vi "do_gsw_step.vi"(6 "Optimisation Resolution":i32, 7 "Sinc Zero":dbl, 11 "Spots In":T1[](array[typedef]) {"Amplitude Correction" step=0.1; "Line Trapping"."Phase Gradient" step=0.05; "Line Trapping"."Vector"."x" step=1e-06 format="%#_6p"; "Line Trapping"."Vector"."y" step=1e-06 format="%#_6p"; "Line Trapping"."Vector"."z" step=1e-06 format="%#_6p"; "NA Position"."r" step=1e-06; "NA Position"."y" step=1e-06; "NA Position"."x" step=1e-06; "Position"."z" step=1e-06; "Position"."y" step=1e-06; "Position"."x" step=1e-06; "Phase" step=0.7753; "Intensity" step=0.1}) -> (1 "non-uniformity":dbl=0.056229799277855076 format="%0.2f", 2 "efficiency":dbl=0.953044464704264, 3 "Spots Out":T1[](array[typedef]) {"Amplitude Correction" step=0.1; "Line Trapping"."Phase Gradient" step=0.05; "Line Trapping"."Vector"."x" step=1e-06 format="%#_6p"; "Line Trapping"."Vector"."y" step=1e-06 format="%#_6p"; "Line Trapping"."Vector"."z" step=1e-06 format="%#_6p"; "NA Position"."r" step=1e-06; "NA Position"."y" step=1e-06; "NA Position"."x" step=1e-06; "Position"."z" step=1e-06; "Position"."y" step=1e-06; "Position"."x" step=1e-06; "Phase" step=0.7753; "Intensity" step=0.1})   [LabVIEW 2010]
uses:
  spot.ctl
  line_trapping.ctl
  <vilib>/Analysis/NI_AALBase.lvlib
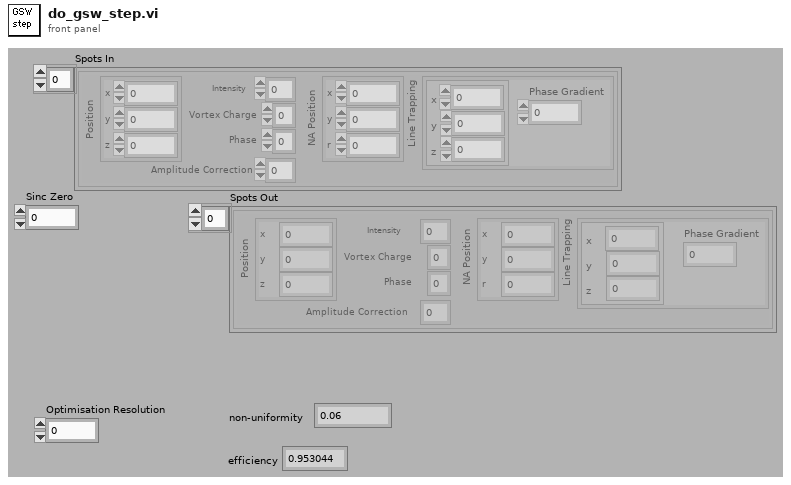
[diagram p1: front panel]
types:
  T1 = typedef "spot.ctl" = cluster{"Position":cluster{"x":dbl, "y":dbl, "z":dbl}, "Intensity":dbl, "Vortex Charge":i8, "Phase":dbl, "NA Position":cluster{"x":dbl, "y":dbl, "r":dbl}, "Line Trapping":T2, "Amplitude Correction":dbl}
  T2 = typedef "line_trapping.ctl" = cluster{"Vector":cluster{"x":dbl, "y":dbl, "z":dbl}, "Phase Gradient":dbl}
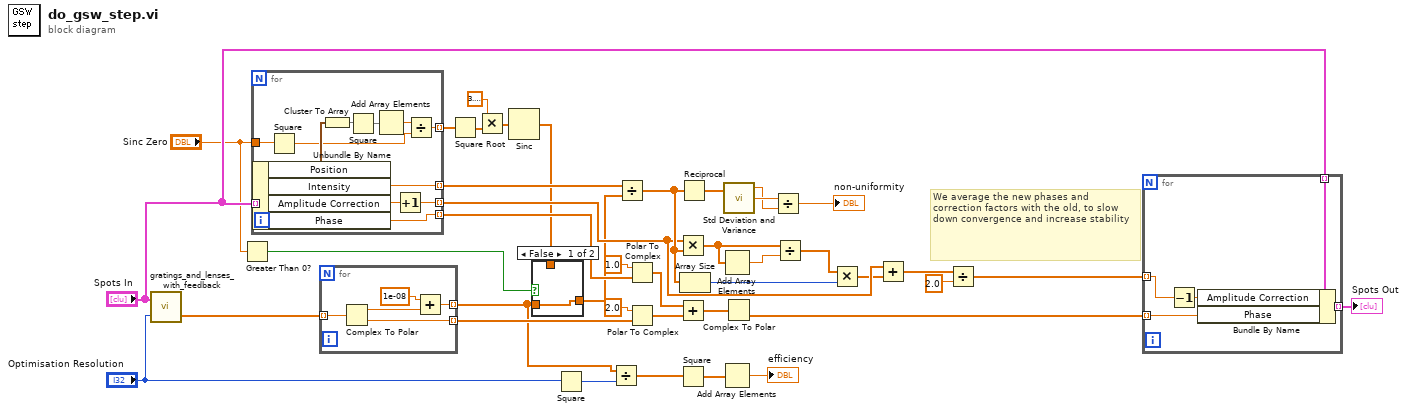
[diagram p0: block diagram]
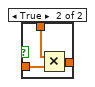
[diagram p2: hidden frame]
diagram:
  # "We average the new phases and correction factors with the old, to slow down convergence and increase stability"
  n1 = call "gratings_and_lenses_with_feedback.vi"("Resolution"="Optimisation Resolution", "Spots 2"="Spots In") -> ("Spot Amplitudes"=w29:cdb[])  [unwired: 1 out]
  n2 = Greater Than 0?(x="Sinc Zero") -> (x > 0?=w2:bool)
  n3 = for {
    tunnel: "Spots In" -> [w52] mode=indexing
    tunnel: [w49] -> w15 mode=indexing
    tunnel: [w48] -> w19 mode=indexing
    tunnel: [w50] -> w31 mode=indexing
    tunnel: "Sinc Zero" -> [w43]
    tunnel: [w41] -> w9 mode=indexing
    n4 = Unbundle By Name(w52) -> ("Position"=w46:cluster{"x":dbl, "y":dbl, "z":dbl}, "Intensity"=w50:dbl, "Amplitude Correction"=w51:dbl, "Phase"=w49:dbl)
    n5 = Square(x=w43) -> (x^2=w42:dbl)
    n6 = Cluster To Array(cluster=w46) -> (array=w45:dbl[])
    n7 = Square(x=w45) -> (x^2=w47:dbl[])
    n8 = Add Array Elements(numeric array=w47) -> (sum=w44:dbl)
    n9 = Increment(x=w51) -> (x+1=w48:dbl)
    n10 = Divide(x=w44, y=w42) -> (x/y=w41:dbl)
  }
  n11 = for {
    tunnel: [w57] -> w16 mode=indexing
    tunnel: [w55] -> w1 mode=indexing
    tunnel: w29 -> [w53] mode=indexing
    n12 = Complex To Polar(r * e^(i*theta)=w53) -> (r=w56:dbl, theta=w57:dbl)
    n13 = Add(x=1e-08, y=w56) -> (x+y=w55:dbl)
  }
  n14 = Square Root(x=w9) -> (sqrt(x)=w8:dbl[])
  n15 = Multiply(x=3.141592653589793, y=w8) -> (x*y=w6:dbl[])
  n16 = Sinc(1:w6) -> (0:w4:dbl[])
  n17 = case shown="False" w2 {
    tunnel: w1 -> [w58 w61]
    tunnel: [w58 w60] -> w5
    tunnel: w4 -> [_ w59]
    frame False {
    }
    frame True {
      n18 = Multiply(x=w59, y=w61) -> (x*y=w60:dbl[])
    }
  }
  n19 = Square(x="Optimisation Resolution") -> (x^2=w22:i32)
  n20 = Divide(x=w1, y=w22) -> (x/y=w21:dbl[])
  n21 = Divide(x=w31, y=w5) -> (x/y=w32:dbl[])
  n22 = Polar To Complex(1:w15, 2:1.0 ("x")) -> (0:w36:cdb[])
  n23 = Polar To Complex(1:w16, 2:2.0 ("x")) -> (0:w37:cdb[])
  n24 = Multiply(x=w19, y=w32) -> (x*y=w13:dbl[])
  n25 = Add(x=w36, y=w37) -> (x+y=w35:cdb[])
  n26 = Square(x=w21) -> (x^2=w20:dbl[])
  n27 = Reciprocal(x=w32) -> (1/x=w33:dbl[])
  n28 = Array Size(array=w32) -> (size(s)=w27:i32)
  n29 = Add Array Elements(numeric array=w13) -> (sum=w12:dbl)
  n30 = Add Array Elements(numeric array=w20) -> (sum=→"efficiency":dbl)
  n31 = call <vilib>:"Std Deviation and Variance.vi"("X"=w33) -> ("mean"=w24:dbl, "standard deviation"=w25:dbl)  [unwired: 1 in, 1 out]
  n32 = Complex To Polar(r * e^(i*theta)=w35) -> (theta=w17:dbl[])  [unwired: 1 out]
  n33 = Divide(x=w25, y=w24) -> (x/y=→"non-uniformity":dbl)
  n34 = Divide(x=w13, y=w12) -> (x/y=w14:dbl[])
  n35 = Multiply(x=w14, y=w27) -> (x*y=w18:dbl[])
  n36 = Add(x=w19, y=w18) -> (x+y=w39:dbl[])
  n37 = Divide(x=w39, y=2.0 ("x")) -> (x/y=w28:dbl[])
  n38 = for {
    tunnel: w28 -> [w65] mode=indexing
    tunnel: w17 -> [w66] mode=indexing
    tunnel: "Spots In" -> [w64] mode=indexing
    tunnel: [w63] -> w10 mode=indexing
    n39 = Decrement(x=w65) -> (x-1=w62:dbl)
    n40 = Bundle By Name(cluster=w64, "Amplitude Correction"=w62, "Phase"=w66) -> (w63:T1)
  }
  "Spots Out" <- w10
